vi "asio_out_in.vi"(8 "Format":cluster{"Rate":i32, "Bits":i32, "Channels":u32}={"Rate"=44100, "Bits"=32, "Channels"=2}, 9 "card #":u32, 10 "data_length":i32, 11 "output data":i32[][](array[numeric])) -> (3 "error play 3":errorcluster)   [LabVIEW 2021]
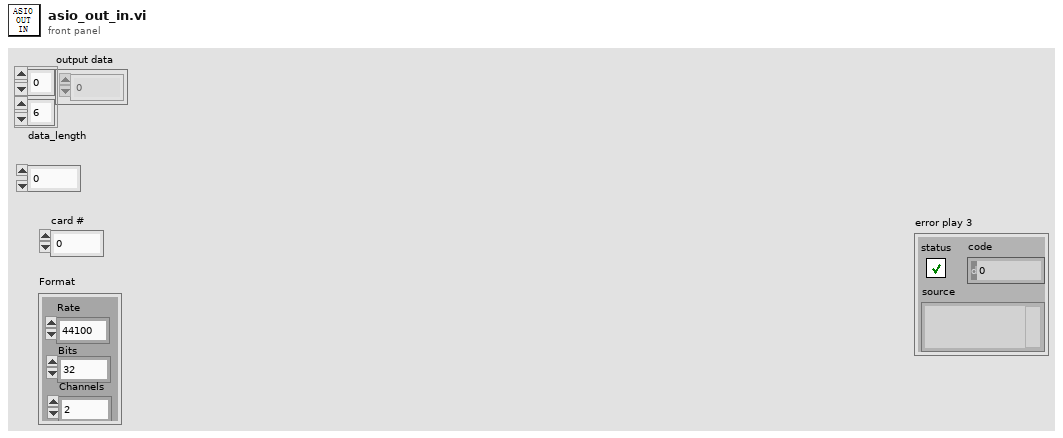
[diagram p1: front panel]
types:
  T1 = cluster{"# buffers":i32, "Buffer size":i32, "unit (ms)":enum16{"time (ms)", "Samples"}}
  T2 = typedef "SoundHandle.ctl" = cluster{"DeviceID":u16, "Samples/buf":u32, "Sampl rate":u32, "Bits/sample":u16, "Channels":u8, "Opened":bool}
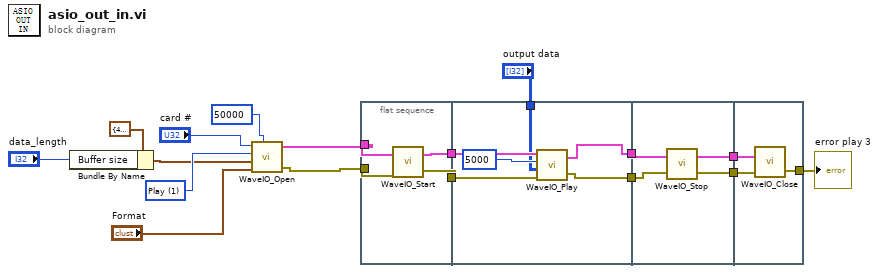
[diagram p0: block diagram]
diagram:
  w11 = u16 1 items=["Record", "Play", "Loopback", "ASIO input", "ASIO output", "Record (WASAPI)", "Play (WASAPI)", "Record Combi", "Play Combi"] ("device type (Record)")
  n1 = Bundle By Name(cluster=T1 {"# buffers"=4, "Buffer size"=88200, "unit (ms)"=enum."Samples"} ("Buffer"), "Buffer size"="data_length") -> (w10:T1)
  n2 = call "WaveIO_Open.vi"("idev"="card #", "Watchdog timeout (msec) (default=OFF)"=50000, "device type (Record)"=w11, "Buffer Config"=w10, "Format (44kHz, 16Bit, stereo)"="Format") -> ("Sound Handle Out"=w4:T2, "error out"=w5:errorcluster)  [unwired: 2 in]
  n3 = flat-sequence {
    tunnel: [w18] -> w17
    tunnel: [w19] -> w16
    tunnel: w5 -> [w21]
    tunnel: w4 -> [w20]
    tunnel: [w24] -> w15
    tunnel: [w22] -> w14
    tunnel: w17 -> [w27]
    tunnel: w16 -> [w26]
    tunnel: "output data" -> [w23]
    tunnel: w15 -> [w31]
    tunnel: w14 -> [w30]
    tunnel: [w29] -> w13
    tunnel: [w28] -> w12
    tunnel: w13 -> [w34]
    tunnel: w12 -> [w33]
    tunnel: [w32] -> w7
    frame #0 {
      n4 = call "WaveIO_Start.vi"("error in (no error)"=w21, "Handle"=w20) -> ("error out"=w19:errorcluster, "Handle Out"=w18:T2)
    }
    frame #1 {
      n5 = call "WaveIO_Play.vi"("error in (no error)"=w26, "data"=w23, "timeout (automatic)"=5000, "Handle"=w27) -> ("error out"=w22:errorcluster, "Handle Out"=w24:T2)
    }
    frame #2 {
      n6 = call "WaveIO_Stop.vi"("error in (no error)"=w30, "Handle"=w31) -> ("error out"=w28:errorcluster, "Handle Out"=w29:T2)
    }
    frame #3 {
      n7 = call "WaveIO_Close.vi"("error in (no error)"=w33, "Handle"=w34) -> ("error out"=w32:errorcluster)  [unwired: 1 out]
    }
  }
  "error play 3" <- w7
